vi "Keithley KE22xx Series Monitor Output.vi"() -> ()   [LabVIEW 2018]
doc: "DESCRIPTION:\n\nThis VI configures the power supply to generate a DC voltage output.\nIt also displays the Output Voltage,Current and Power as per the selected parameter. \n\nINSTRUCTIONS:\n1. Enter the resource name.\n2. Select the desired Channel.\n3. Enter voltage or current value to set the voltage or current value of the power supply .\n4. Set On/Off switch to Enable if you want the generated voltage to appear at the instrument's output. \n5. Select Local/Remote mode operation.If local command is select ,this will set the instrument in local mode.\n6.Select the parameter from the control,to read the responce from the instrument.\n7.Run the VI.\n\nNOTES:\nNotice the order of the power supply component VIs in the block diagram. The first VI in a sequence is the power supply Initialize.vi, which provides a VISA session to the instrument driver. The last VI in a sequence must be the power supply Close.vi which closes the Visa session."
uses:
  Keithley KE22xx Series.lvlib
panel:
  in  "Channel Select":enum16{"Channel 1", "Channel 2", "Channel 3"}(ring)
  in  "Measurement Function(0:Voltage)":u16(ring) items=["Voltage", "Current", "Power"]
  in  "Function(0:Voltage)":u16(ring) items=["Voltage", "Current"]
  in  "Control Mode(1:Remote)":u16(ring)=1 items=["Local", "Remote"]
  in  "Manual Range(0.00)":dbl format="%.2f"
  in  "Enable Output (T: Enable)":bool=TRUE
  in  "Unit(V)":u16(ring) items=["V", "mV", "kV", "A", "mA"]
  out "Measurement":string
  in  "VISA resource name":refnum<visa-resource-name>
  # "© 2012 Keithley Instruments, Inc. ALL RIGHTS RESERVED"
  # "Configure Instrument"
  # "Read Measurement"
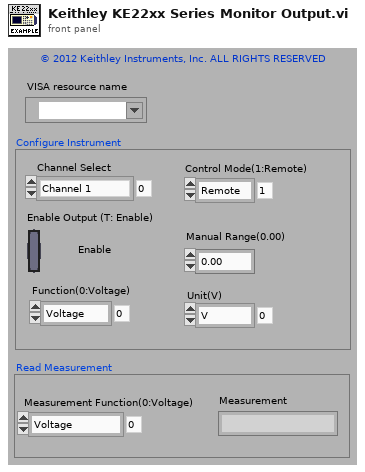
[diagram p1: front panel]
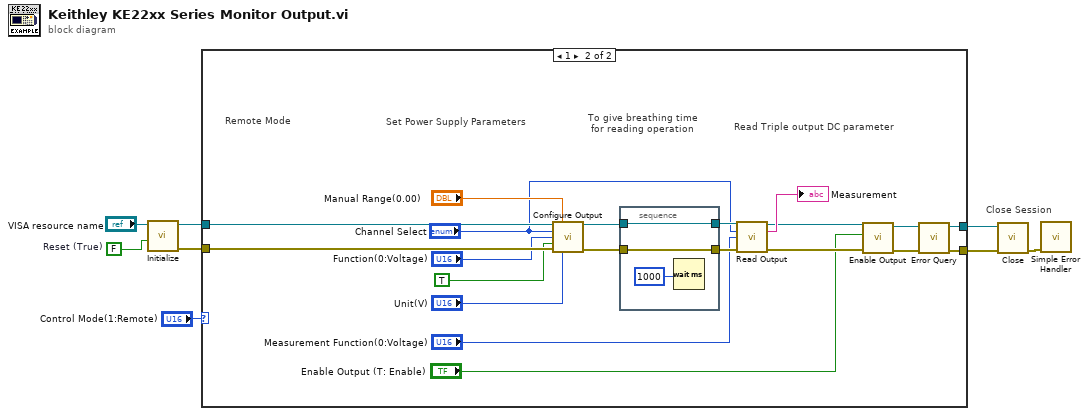
[diagram p0: block diagram]
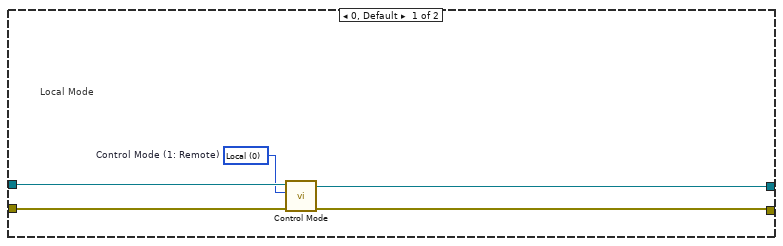
[diagram p2: hidden frame]
diagram:
  w1 = FALSE items=["OFF", "ON", "OFF", "ON"]  # Reset (True)
  # "Close Session"
  n1 = call "Initialize.vi"("Reset (True)"=w1, "VISA resource name"="VISA resource name") -> ("error out"=w2:errorcluster, "VISA resource name out"=w3:refnum<visa-resource-name>)  [unwired: 8 in]
  n2 = case shown="1" "Control Mode(1:Remote)" {
    tunnel: [w10 w24] -> w4
    tunnel: w3 -> [w13 w29]
    tunnel: w2 -> [w12 w28]
    tunnel: [w9 w25] -> w6
    frame 0, Default {
      w11 = u16 0 items=["Local", "Remote", "Remote Lock"]  # Control Mode (1: Remote)
      # "Local Mode"
      n3 = call "Control Mode.vi"("error in (no error)"=w12, "Control Mode (1: Remote)"=w11, "VISA resource name"=w13) -> ("error out"=w10:errorcluster, "VISA resource name out"=w9:refnum<visa-resource-name>)  [unwired: 7 in]
    }
    frame 1 {
      # "Read Triple output DC parameter"
      # "To give breathing time\n for reading operation"
      # "Set Power Supply Parameters"
      # "Remote Mode"
      n4 = call "Configure Output.vi"("VISA resource name"=w29, "Manual Range(0.00)"="Manual Range(0.00)", "Channel Select"="Channel Select", "Function(0:Voltage)"="Function(0:Voltage)", "Enable Output (T: Enable)"=TRUE, "error in (no error)"=w28, "Unit(V)"="Unit(V)") -> ("VISA resource name out"=w33:refnum<visa-resource-name>, "error out"=w31:errorcluster)  [unwired: 7 in]
      n5 = stacked-sequence {
        tunnel: w33 -> [w35]
        tunnel: [w35] -> w32
        tunnel: w31 -> [w34]
        tunnel: [w34] -> w30
        frame #0 {
          n6 = Wait (ms)(milliseconds to wait=u32 1000 ("millisecond multiple")) -> ()  [unwired: 1 out]
        }
      }
      n7 = call "Read Output.vi"("VISA resource name"=w32, "Channel Select"="Channel Select", "Measurement Function (0:Voltage)"="Measurement Function(0:Voltage)", "error in (no error)"=w30) -> ("VISA resource name out"=w18:refnum<visa-resource-name>, "Measurement"=→"Measurement":string, "error out"=w16:errorcluster)  [unwired: 9 in]
      n8 = call "Enable Output.vi"("error in (no error)"=w16, "Enable Output (T: Enable)"="Enable Output (T: Enable)", "VISA resource name"=w18) -> ("error out"=w15:errorcluster, "VISA resource name out"=w17:refnum<visa-resource-name>)  [unwired: 7 in]
      n9 = call "Error Query.vi"("error in (no error)"=w15, "VISA resource name"=w17) -> ("error out"=w24:errorcluster, "VISA resource name out"=w25:refnum<visa-resource-name>)  [unwired: 6 in, 2 out]
    }
  }
  n10 = call "Close.vi"("error in (no error)"=w4, "VISA resource name"=w6) -> ("error out"=w5:errorcluster)  [unwired: 9 in]
  n11 = call <vilib>:"Simple Error Handler.vi"("error in (no error)"=w5) -> ()  [unwired: 1 in, 8 out]
